vi "Init Device.vi"(8 "error in (no error)":errorcluster, 11 "niDigital in":refnum<class "niDigital.lvclass">) -> (0 "error out":errorcluster, 3 "niDigital out":refnum<class "niDigital.lvclass">)   [LabVIEW 2020, in "niDigital.lvclass"]
uses:
  niDigital.lvclass
  <instrlib>/niDigital/niDigital.llb/niDigital Load Specifications Levels and Timing (Single).vi
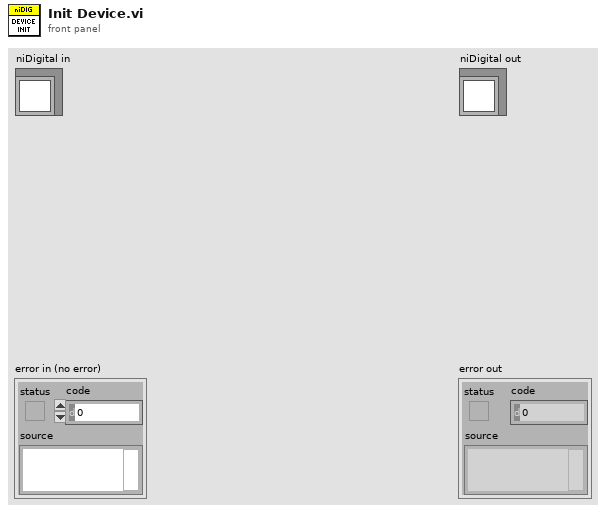
[diagram p1: front panel]
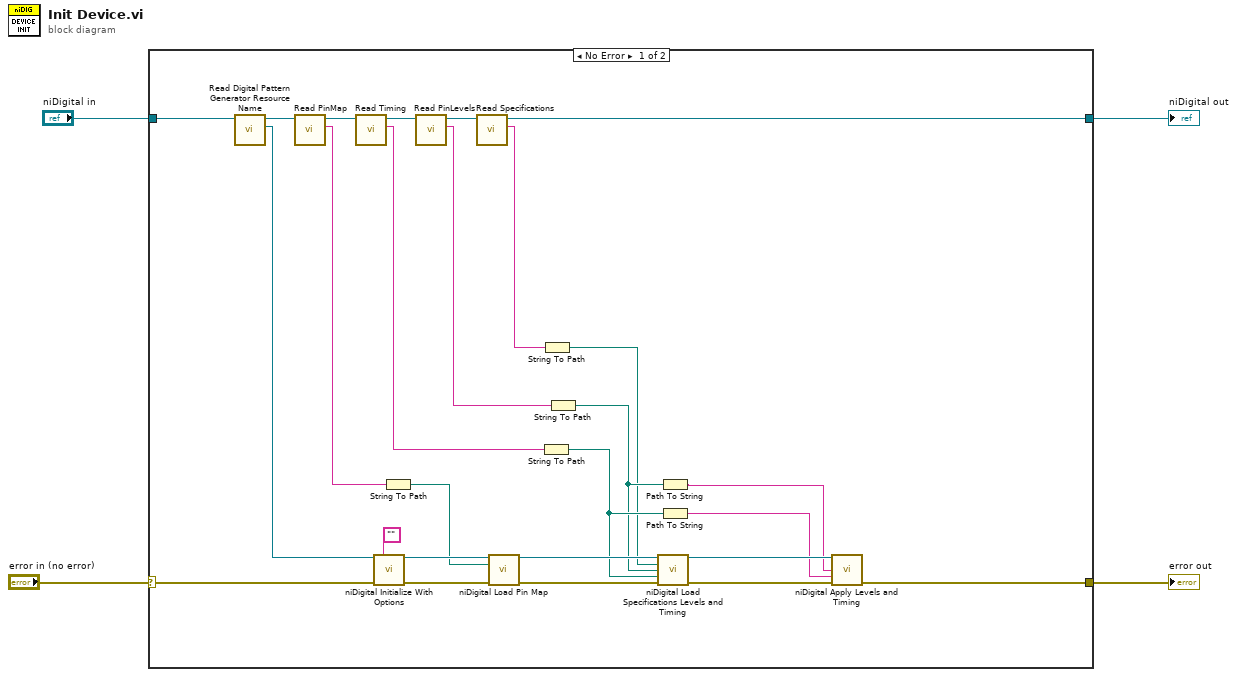
[diagram p0: block diagram]
diagram:
  n1 = case shown="No Error" "error in (no error)" {
    selector: "error in (no error)" -> [w18 w31]
    tunnel: [w16 w31] -> w3
    tunnel: "niDigital in" -> [w15 w32]
    tunnel: [w5 w32] -> w1
    frame No Error {
      n2 = call-dynamic "Read Digital Pattern Generator Resource Name.vi"("niDigital in"=w15) -> ("Digital Pattern Generator Resource Name"=w17:refnum<k15>, "niDigital out"=w9:refnum<class "niDigital.lvclass">)  [unwired: 9 in]
      n3 = call-dynamic "Read PinMap.vi"("niDigital in"=w9) -> ("PinMap"=w14:string, "niDigital out"=w8:refnum<class "niDigital.lvclass">)  [unwired: 9 in]
      n4 = call-dynamic "Read Timing.vi"("niDigital in"=w8) -> ("Timing"=w12:string, "niDigital out"=w7:refnum<class "niDigital.lvclass">)  [unwired: 9 in]
      n5 = call <instrlib>:"niDigital Initialize With Options.vi"("resource name"=w17, "option string"="", "error in"=w18) -> ("instrument handle"=w30:refnum<k15>, "error out"=w29:errorcluster)  [unwired: 11 in]
      n6 = String To Path(string=w14) -> (path=w13:path)
      n7 = call-dynamic "Read PinLevels.vi"("niDigital in"=w7) -> ("PinLevels"=w11:string, "niDigital out"=w6:refnum<class "niDigital.lvclass">)  [unwired: 9 in]
      n8 = call-dynamic "Read Specifications.vi"("niDigital in"=w6) -> ("Specifications"=w10:string, "niDigital out"=w5:refnum<class "niDigital.lvclass">)  [unwired: 9 in]
      n9 = call <instrlib>:"niDigital Load Pin Map.vi"("instrument handle"=w30, "pin map file"=w13, "error in"=w29) -> ("instrument handle out"=w28:refnum<k15>, "error out"=w27:errorcluster)  [unwired: 11 in]
      n10 = String To Path(string=w12) -> (path=w26:path)
      n11 = String To Path(string=w10) -> (path=w24:path)
      n12 = String To Path(string=w11) -> (path=w25:path)
      n13 = call-poly <instrlib>:"niDigital Load Specifications Levels and Timing.vi"("instrument handle"=w28, "specifications file path"=w24, "levels file path"=w25, "timing file path"=w26, "error in"=w27) -> ("instrument handle out"=w22:refnum<k15>, "error out"=w21:errorcluster)  [unwired: 9 in]
      n14 = Path To String(path=w25) -> (string=w20:string)
      n15 = Path To String(path=w26) -> (string=w19:string)
      n16 = call <instrlib>:"niDigital Apply Levels and Timing.vi"("instrument handle"=w22, "levels sheet"=w20, "timing sheet"=w19, "error in"=w21) -> ("error out"=w16:errorcluster)  [unwired: 10 in, 1 out]
    }
    frame Error {
    }
  }
  "error out" <- w3
  "niDigital out" <- w1
